vi "Report Get-Resort Group Data.vi"(11 "Array in":string[][](array[string])) -> (1 "values":variant[](array[variant]), 2 "Array out":string[][](array[string]), 3 "Array 3":string[][](array[string]), 5 "Channels":i32)   [LabVIEW 2020, in "Report.lvlib"]
uses:
  Report.lvlib
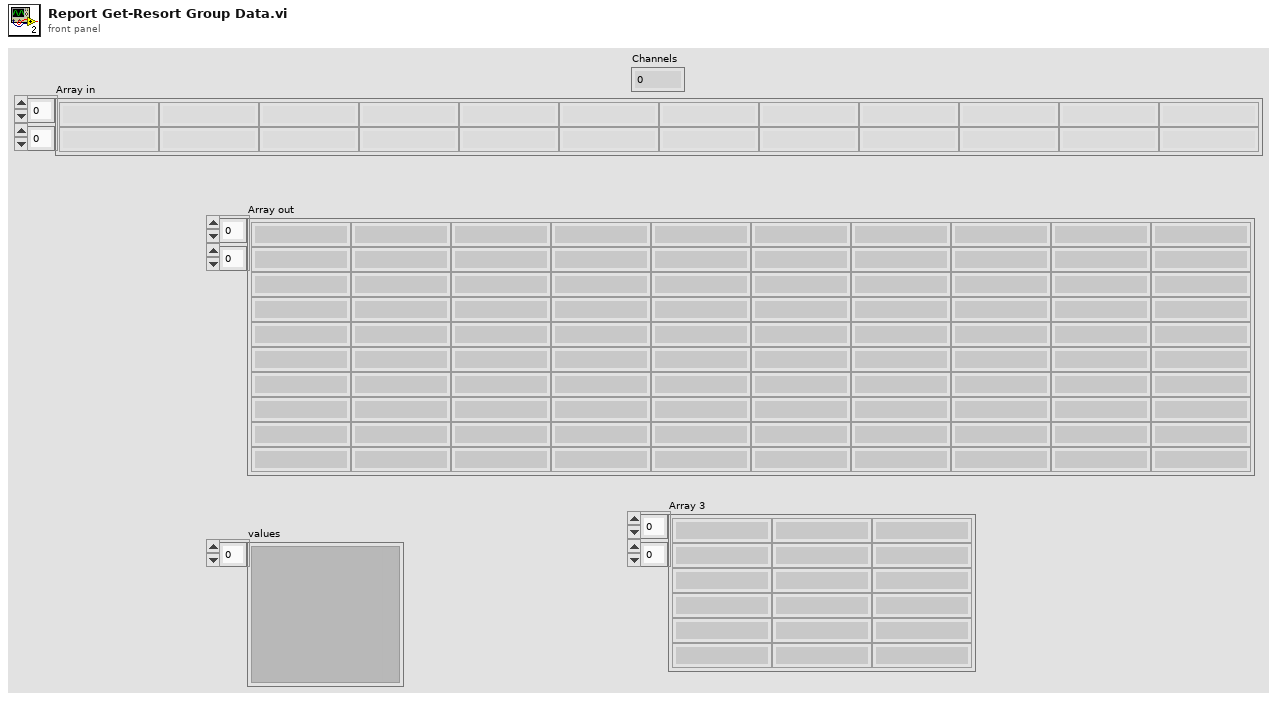
[diagram p1: front panel]
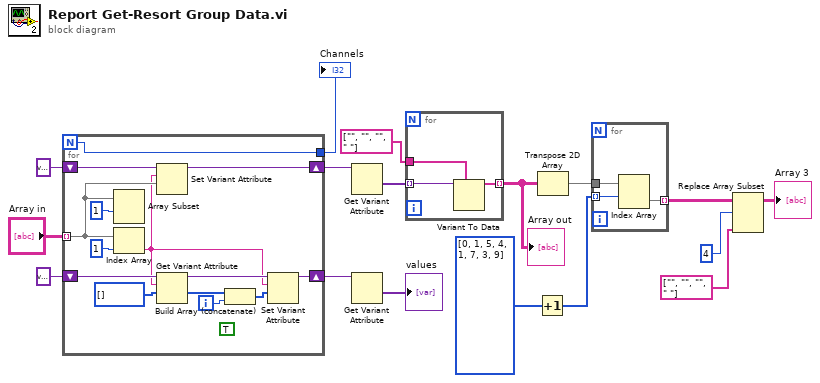
[diagram p0: block diagram]
diagram:
  n1 = for {
    N -> [w18]
    tunnel: "Array in" -> [w27] mode=indexing
    shift-right: [w30] -> w12
    shift-left: variant -> [w31]
    shift-right: [w20] -> w16
    shift-left: variant -> [w26]
    tunnel: [w18] -> w3
    i -> [w19]
    (unwired) TRUE ("border? (F)")
    n2 = Array Subset(array=w27, index=1) -> ()  [unwired: 1 in, 1 out]
    n3 = Index Array(array=w27, index=1) -> (element=w22:string)
    n4 = Set Variant Attribute(Variant=w31, name=w22, value=w27) -> (Variant out=w30:variant)  [unwired: 1 in, 2 out]
    n5 = Get Variant Attribute(Variant=w26, name=w22, default value (empty Variant)=i32[] [] ("index (row)")) -> (duplicate Variant=w23:variant, value=w24:i32[])  [unwired: 1 in, 2 out]
    n6 = Build Array (concatenate)(w24, w19) -> (w21:i32[])
    n7 = Set Variant Attribute(Variant=w23, name=w22, value=w21) -> (Variant out=w20:variant)  [unwired: 1 in, 2 out]
  }
  "Channels" <- w3
  n8 = Get Variant Attribute(Variant=w12) -> (values=w13:variant[])  [unwired: 3 in, 3 out]
  n9 = Get Variant Attribute(Variant=w16) -> (values=→"values":variant[])  [unwired: 3 in, 3 out]
  n10 = for {
    tunnel: w13 -> [w34] mode=indexing
    tunnel: string[] ["", "", "", " "] ("new element/subarray") -> [w33]
    tunnel: [w32] -> w15 mode=indexing
    n11 = Variant To Data(type=w33, Variant=w34) -> (data=w32:string[])  [unwired: 1 in, 1 out]
  }
  "Array out" <- w15
  n12 = Increment(x=i32[] [0, 1, 5, 4, 1, 7, 3, 9] ("index (row)")) -> (x+1=w9:i32[])
  n13 = Transpose 2D Array(2D array=w15) -> (transposed array=w4:string[][])
  n14 = for {
    tunnel: w4 -> [w37]
    tunnel: w9 -> [w36] mode=indexing
    tunnel: [w35] -> w5 mode=indexing
    n15 = Index Array(array=w37, index (row)=w36) -> (element=w35:string[])  [unwired: 1 in]
  }
  n16 = Replace Array Subset(array=w5, new element=string[] ["", "", "", " "] ("new element/subarray"), index (row)=4) -> (→"Array 3":string[][])  [unwired: 1 in]
